vi "LvHostsEdit4cRIO_SUB_Login_Dialog.vi"(7 "host in":string, 10 "password in":string, 11 "userID in":string) -> (1 "Cancel?":bool, 2 "password out":string, 3 "userID out":string, 5 "host out":string)   [LabVIEW 2014]
panel:
  in  "Btn Cancel":bool
  in  "Btn OK":bool
  in  "IP":string caption="IP or hostname:"
  in  "password":string caption="password:"
  in  "userID":string="admin" caption="userID:"
  out "/etc/hosts uri":string
  # "IP or hostname"
  # "cRIOのIP, userID, passwordを入力してください。"
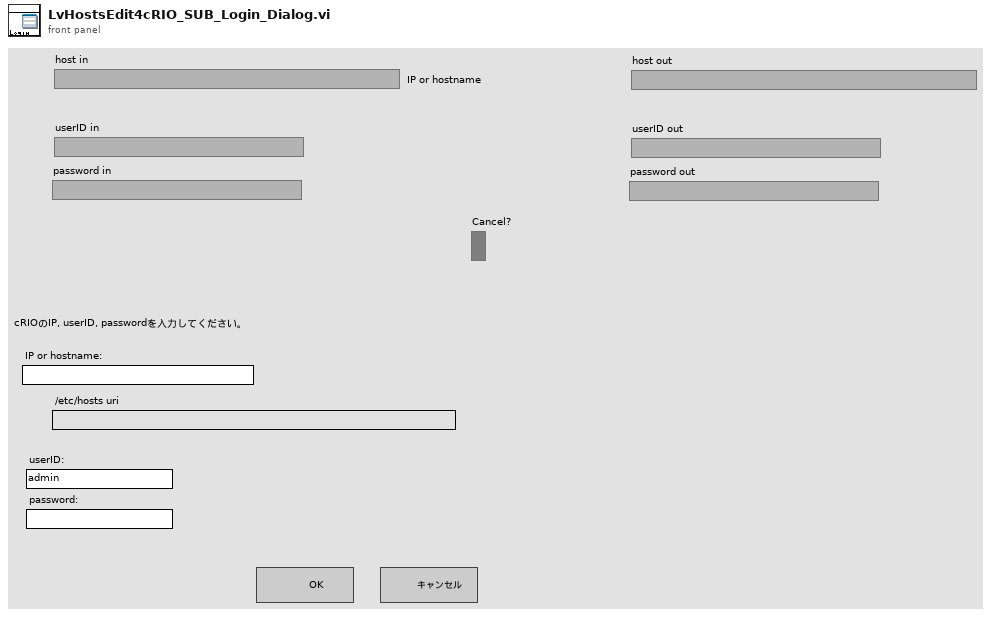
[diagram p1: front panel]
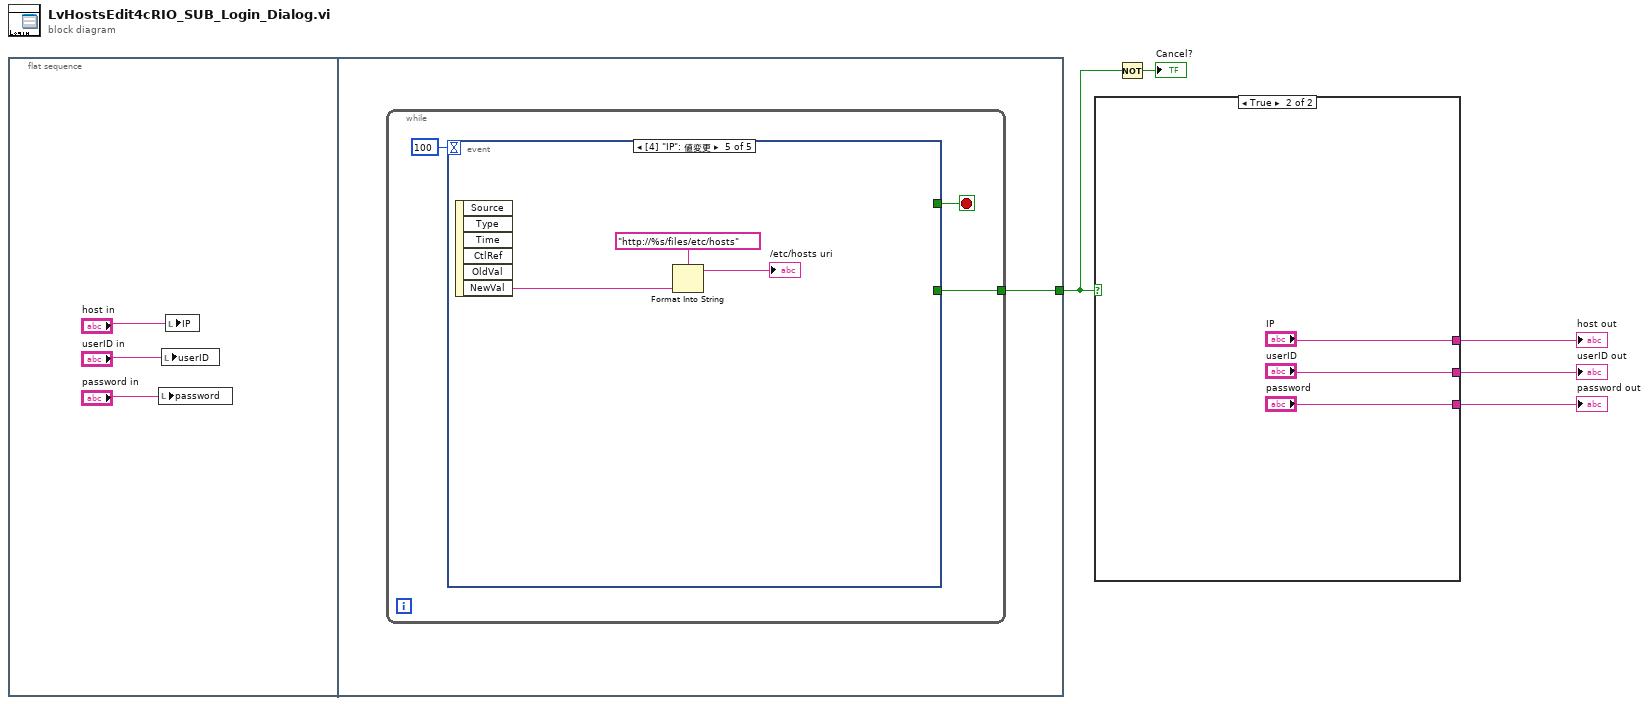
[diagram p0: block diagram]
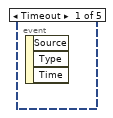
[diagram p3: hidden frame]
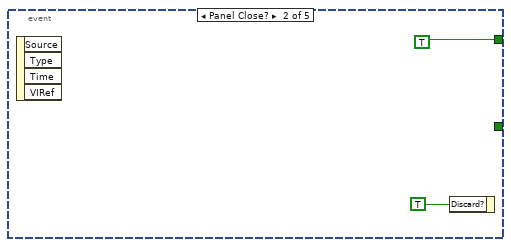
[diagram p4: hidden frame]
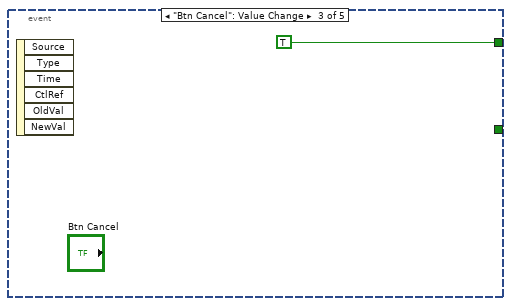
[diagram p5: hidden frame]
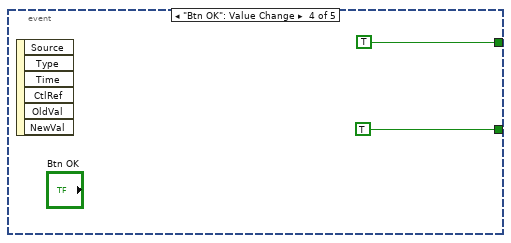
[diagram p6: hidden frame]
diagram:
  n1 = flat-sequence {
    tunnel: [w9] -> w5
    frame #0 {
      n2 = local write "password"("password in") -> ()
      n3 = local write "userID"("userID in") -> ()
      n4 = local write "IP"("host in") -> ()
    }
    frame #1 {
      n5 = while {
        tunnel: [w10] -> w9
        stop <- w11 stop-if-true
        n6 = event shown="[4] \"IP\": 値変更" {
          selector: _ -> [_ _ _ _ _]
          dyn-events: _ -> [_ _ _ _ _]
          timeout: 100 -> [_ _ _ _ _]
          tunnel: [_ TRUE TRUE TRUE _] -> w11
          tunnel: [_ _ _ TRUE _] -> w10
          event Timeout {
            n7 = event-data() -> ()  [unwired: 1 in, 3 out]
          }
          event Panel Close? {
            n8 = event-data() -> ()  [unwired: 1 in, 4 out]
            n9 = event-data("Discard?"=TRUE ("破棄?")) -> ()  [unwired: 1 in, 1 out]
          }
          event "Btn Cancel": Value Change {
            n10 = event-data() -> ()  [unwired: 1 in, 6 out]
          }
          event "Btn OK": Value Change {
            n11 = event-data() -> ()  [unwired: 1 in, 6 out]
          }
          event "IP": Value Change {
            n12 = event-data() -> ("NewVal"=w18:string)  [unwired: 1 in, 5 out]
            n13 = Format Into String(format string="http://%s/files/etc/hosts", w18) -> (resulting string=→"/etc/hosts uri":string)  [unwired: 2 in, 1 out]
          }
        }
      }
    }
  }
  n14 = case shown="TRUE" w5 {
    tunnel: [_ "IP"] -> w3
    tunnel: [_ "userID"] -> w2
    tunnel: [_ "password"] -> w1
    frame False {
    }
    frame True {
    }
  }
  "host out" <- w3
  "userID out" <- w2
  "password out" <- w1
  n15 = Not(x=w5) -> (.not. x?=→"Cancel?":bool)
